vi "Initialize Stream.vi"(8 "error in (no error)":errorcluster, 11 "Channel GUI in":refnum<class "Channel.lvclass">) -> (0 "error out":errorcluster, 3 "Channel GUI out":refnum<class "Channel.lvclass">)   [LabVIEW 2018, in "Channel.lvclass"]
uses:
  Channel.lvclass
  Channel.lvclass/Channel.ctl
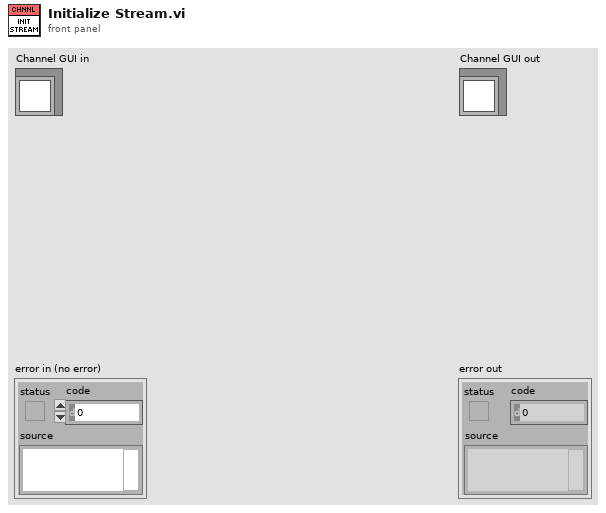
[diagram p1: front panel]
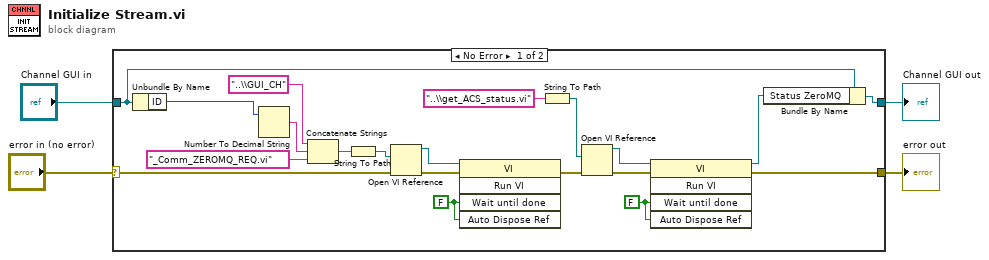
[diagram p0: block diagram]
diagram:
  n1 = case shown="No Error" "error in (no error)" {
    selector: "error in (no error)" -> [w15 w26]
    tunnel: [w7 w26] -> w4
    tunnel: [w21 w25] -> w3
    tunnel: "Channel GUI in" -> [w22 w25]
    frame No Error {
      w10 = FALSE ("Wait Until Done")
      w23 = FALSE ("Wait Until Done")
      n2 = Unbundle By Name(w22) -> ("ID"=w19:u8)
      n3 = Number To Decimal String(number=w19) -> (decimal integer string=w16:string)  [unwired: 1 in]
      n4 = Concatenate Strings("..\\GUI_CH" ("name or relative path"), w16, "_Comm_ZEROMQ_REQ.vi" ("name or relative path")) -> (w17:string)
      n5 = String To Path(string=w17) -> (path=w18:path)
      n6 = Open VI Reference(vi path=w18, error in (no error)=w15) -> (vi reference=w24:refnum<vi>, error out=w20:errorcluster)  [unwired: 4 in]
      n7 = invoke class="VI" method="Run VI"(reference=w24, error in=w20, "Wait until done"=w23, "Auto Dispose Ref"=w23) -> (error out=w8:errorcluster)  [unwired: 1 in, 4 out]
      n8 = String To Path(string="..\\get_ACS_status.vi" ("name or relative path")) -> (path=w12:path)
      n9 = Open VI Reference(vi path=w12, error in (no error)=w8) -> (vi reference=w9:refnum<vi>, error out=w11:errorcluster)  [unwired: 4 in]
      n10 = invoke class="VI" method="Run VI"(reference=w9, error in=w11, "Wait until done"=w10, "Auto Dispose Ref"=w10) -> (reference out=w6:refnum<vi>, error out=w7:errorcluster)  [unwired: 1 in, 3 out]
      n11 = Bundle By Name(cluster=w22, "Status ZeroMQ"=w6) -> (w21:refnum<class "Channel.lvclass">)
    }
    frame Error {
    }
  }
  "error out" <- w4
  "Channel GUI out" <- w3
